vi "svl_Clip to Baseline (autoscale).vi"(0 "waterfall data":dbl[][](array[numeric]) format="%.2f", 1 "baseline":dbl format="%.2f") -> (2 "clipped data":dbl[][](array[numeric]) format="%.2f", 3 "z autoscale":cluster{"z min":dbl, "z max":dbl} {"z max" format="%.2f"; "z min" format="%.2f"}, 4 "z scale":cluster{"z min":dbl, "z max":dbl} {"z max" format="%.2f"; "z min" format="%.2f"})   [LabVIEW 2017]
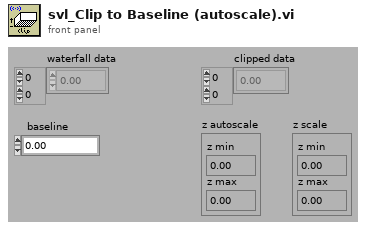
[diagram p1: front panel]
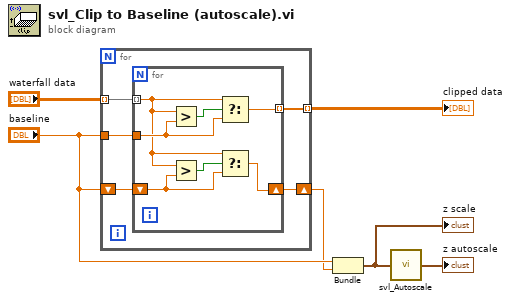
[diagram p0: block diagram]
diagram:
  n1 = for {
    tunnel: "waterfall data" -> [w9] mode=indexing
    tunnel: "baseline" -> [w11]
    tunnel: [w10] -> w6 mode=indexing
    shift-right: [w7] -> w3
    shift-left: "baseline" -> [w8]
    n2 = for {
      tunnel: w9 -> [w14] mode=indexing
      tunnel: w11 -> [w17]
      tunnel: [w16] -> w10 mode=indexing
      shift-right: [w12] -> w7
      shift-left: w8 -> [w13]
      n3 = Greater?(x=w14, y=w17) -> (0:w18:bool)
      n4 = Greater?(x=w14, y=w13) -> (0:w15:bool)
      n5 = Select(t=w14, s=w18, f=w17) -> (s? t:f=w16:dbl)
      n6 = Select(t=w14, s=w15, f=w13) -> (s? t:f=w12:dbl)
    }
  }
  "clipped data" <- w6
  n7 = Bundle("baseline"="baseline", "baseline"=w3) -> (w1:cluster{"baseline":dbl, "baseline":dbl})  [unwired: 1 in]
  "z scale" <- w1
  n8 = call <vilib>:"svl_Autoscale.vi"("scale"=w1) -> ("autoscale"=→"z autoscale":cluster{"min":dbl, "max":dbl})
